vi "WPI_CANTalonSRX_Open.vi"(6 "Invert":bool, 8 "error in":errorcluster, 9 "Master Device Number":u8, 10 "Device Number":u8, 11 "Control Mode":T1) -> (0 "error out":errorcluster, 3 "CAN Talon SRX Ref":T2={"DeviceStatus"={"status"=FALSE, "code"=0, "source"=""}, "Type"=enum."PWM", "PWM"={"PWM Channel"=enum."PWM 1", "DeadBand"={"Name"="", "maxPositivePwm"=0, "minPositivePwm"=0, "centerPwm"=0, "maxNegativePwm"=0, "minNegativePwm"=0, "angularRange"=0}}, "CAN"={"Device Number"=0, "SetOutput VI Ref"=variant(enum8{"Percent VBus", "Current", "Speed", "Position", "Voltage"} enum."Percent VBus"), "GetOutput VI Ref"=variant(refnum<k1> refnum), "Enable VI Ref"=variant(dbl 12.0), "Disable VI Ref"=variant(enum8{"Percent VBus", "Speed", "Position", "Slave", "Unchanged / Invalid", "Voltage Compensation", "Current", "Motion Profile"} enum."Percent VBus"), "Data"=variant}, "Invert"=FALSE})   [LabVIEW 2016]
doc: "Read status information from a CAN Jaguar.\n\nThis VI allows you to specify which parts of the status you care about so that you do not waste CAN bus bandwidth. Use this VI to read status <B>On Demand</B> or status that is already received on a <B>Periodic Status Channel</B>.\n\nAll outputs are in engineering units (Volts, Amps, degrees Celsius, Rotations, and Rotations per Minute)\n\nSticky outputs are faults or limits that have occurred since the last time they were read, but may not be the current condition."
uses:
  <vilib>/Rock Robotics/WPI/MotorControl/WPI_MotorControlDeviceRef.ctl
  <vilib>/Rock Robotics/WPI/MotorControl/WPI_MotorControlType.ctl
  <vilib>/Rock Robotics/SystemInterfaces/DIO/FPGA_DIOPWMChannel.ctl
  <vilib>/Rock Robotics/WPI/PWM/WPI_PWMDeadband.ctl
  WPI_CANTalonSRX_APIControlMode.ctl
  WPI_CANTalonSRX_GlobalOps.ctl
  <vilib>/Rock Robotics/SystemInterfaces/NetworkCommunication/NetComm_UsageReport_ResourceType.ctl
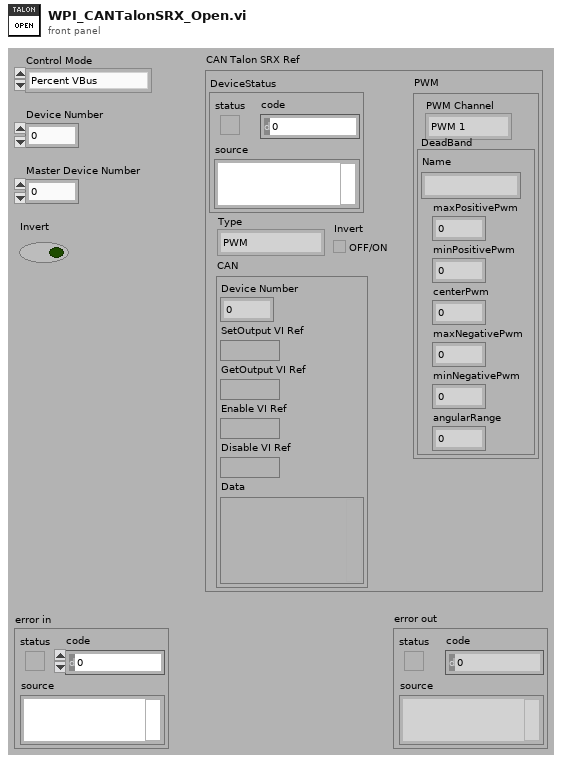
[diagram p1: front panel]
types:
  T1 = typedef "WPI_CANTalonSRX_APIControlMode.ctl" = enum8{"Percent VBus", "Speed", "Position", "Slave", "Unchanged / Invalid", "Voltage Compensation", "Current", "Motion Profile", "Motion Magic"}
  T2 = typedef "WPI_MotorControlDeviceRef.ctl" = cluster{"DeviceStatus":errorcluster, "Type":T3, "PWM":cluster{"PWM Channel":T4, "DeadBand":T5}, "CAN":cluster{"Device Number":u8, "SetOutput VI Ref":variant, "GetOutput VI Ref":variant, "Enable VI Ref":variant, "Disable VI Ref":variant, "Data":variant}, "Invert":bool}
  T3 = typedef "WPI_MotorControlType.ctl" = enum16{"PWM", "CAN"}
  T4 = typedef "FPGA_DIOPWMChannel.ctl" = enum8{"PWM 0", "PWM 1", "PWM 2", "PWM 3", "PWM 4", "PWM 5", "PWM 6", "PWM 7", "PWM 8", "PWM 9", "PWM MXP 0", "PWM MXP 1", "PWM MXP 2", "PWM MXP 3", "PWM MXP 4", "PWM MXP 5", "PWM MXP 6", "PWM MXP 7", "PWM MXP 8", "PWM MXP 9", "Invalid"}
  T5 = typedef "WPI_PWMDeadband.ctl" = cluster{"Name":string, "maxPositivePwm":i32, "minPositivePwm":i32, "centerPwm":i32, "maxNegativePwm":i32, "minNegativePwm":i32, "angularRange":u16}
  T6 = typedef "WPI_CANTalonSRX_GlobalOps.ctl" = enum16{"Read For Send", "Write After Receive General", "Write After Receive Feedback", "Write After Receive Encoder", "Write After Receive Ain", "Write Error", "Get All", "Set Output", "Set Mode", "Set Master ID", "Set Brake Mode", "Set Reverse Feedback Sensor", "Set Reverse Closed Loop Output", "Set Override Limits", "Set Forward Limit Enabled", "Set Reverse Limit Enabled", "Set Feedback Select", "Set Profile Select", "Set Throttle Ramp Rate", "Disable", "Set Enc Codes Per Rev", "Set Num Pot Turns", "Set Control Frame Rate", "Enable Legacy Control", "Write After Receive Pulse Width", "Set Enable Frame Rate", "Write After Receive Motion Profile", "Set Motion Profile Flow Control", "Set Motion Profile Control Frame Rate", "Set Current Limit Enable"}
  T7 = typedef "NetComm_UsageReport_ResourceType.ctl" = enum8{"Controller", "Module", "Language", "CANPlugin", "Accelerometer", "ADXL345", "AnalogChannel", "AnalogTrigger", "AnalogTriggerOutput", "CANJaguar", "Compressor", "Counter", "Dashboard", "DigitalInput", "DigitalOutput", "DriverStationCIO", "DriverStationEIO", "DriverStationLCD", "Encoder", "GearTooth", "Gyro", "I2C", "Framework", "Jaguar", "Joystick", "Kinect", "KinectStick", "PIDController", "Preferences", "PWM", "Relay", "RobotDrive", "SerialPort", "Servo", "Solenoid", "SPI", "Task", "Ultrasonic", "Victor", "Button", "Command", "AxisCamera", "PCVideoServer", "SmartDashboard", "Talon", "HiTechnicColorSensor", "HiTechnicAccel", "HiTechnicCompass", "SRF08", "AnalogOutput", "Victor SP", "Talon SRX", "CAN Talon SRX", "ADXL362 Accel", "ADXRS450 Gyro", "Rev SPARK", "Mindsensors SD540", "Digital Filter", "ADIS16448", "PDP", "PCM", "PigeonIMU"}
  T8 = cluster{"Control Mode":T1, "Encoder Initial Position":dbl, "MaxVout":dbl}
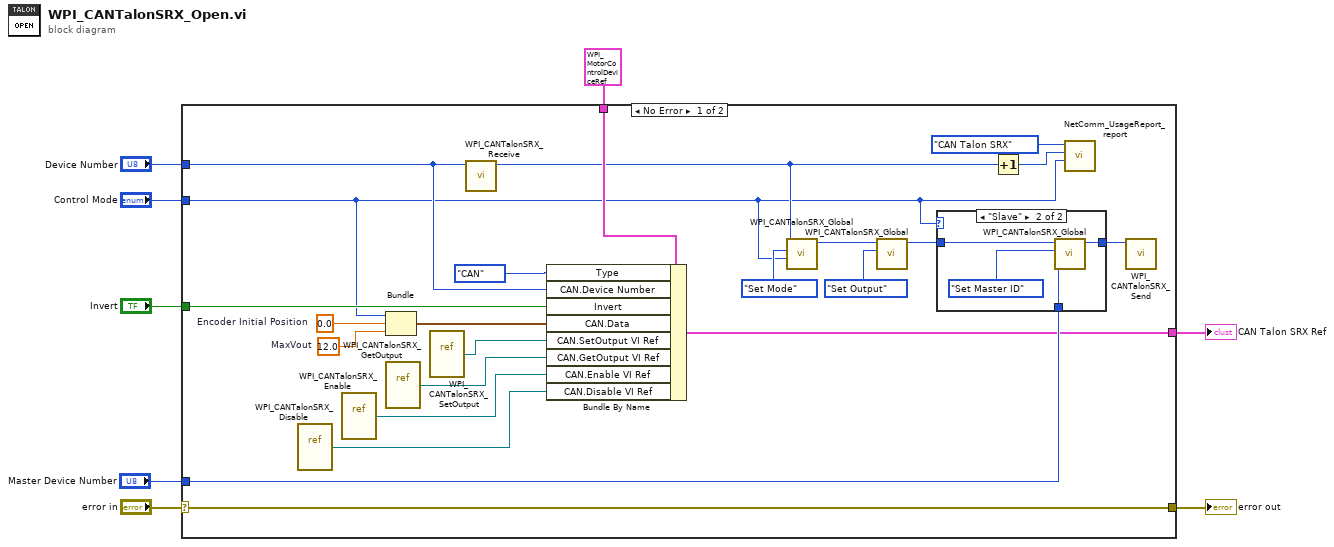
[diagram p0: block diagram]
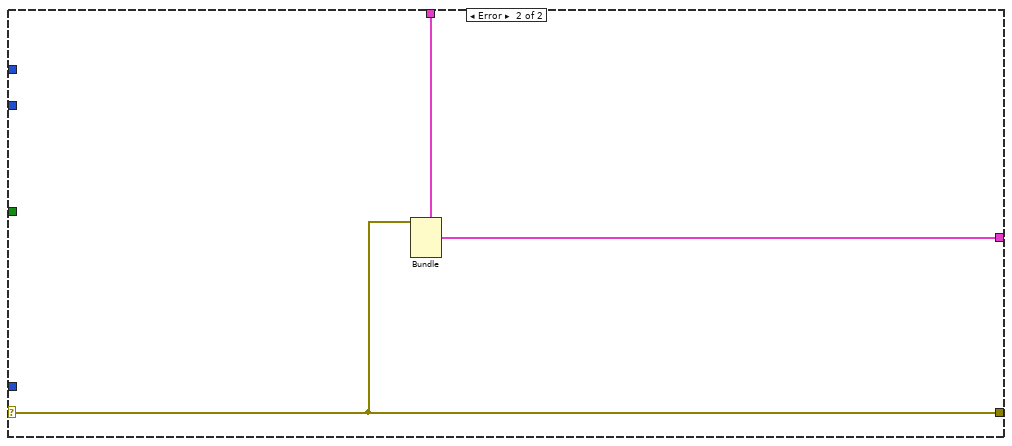
[diagram p3: hidden frame]
diagram:
  n1 = case shown="No Error" "error in" {
    selector: "error in" -> [w14 w37]
    tunnel: [w14 w37] -> w8
    tunnel: "Invert" -> [w22 _]
    tunnel: T2 {"DeviceStatus"={"status"=FALSE, "code"=0, "source"=""}, "Type"=enum."CAN", "PWM"={"PWM Channel"=enum."PWM 1", "DeadBand"={"Name"="", "maxPositivePwm"=0, "minPositivePwm"=0, "centerPwm"=0, "maxNegativePwm"=0, "minNegativePwm"=0, "angularRange"=0}}, "CAN"={"Device Number"=0, "SetOutput VI Ref"=variant(refnum<vi> refnum), "GetOutput VI Ref"=variant(refnum<vi> refnum), "Enable VI Ref"=variant(refnum<vi> refnum), "Disable VI Ref"=variant(refnum<vi> refnum), "Data"=variant(cluster{"Control Mode":enum8{"Percent VBus", "Speed", "Position", "Slave", "Unchanged / Invalid", "Voltage Compensation", "Current", "Motion Profile"}, "Encoder Initial Position":dbl, "MaxVout":dbl} {"Control Mode"=enum."Percent VBus", "Encoder Initial Position"=0.0, "MaxVout"=12.0})}, "Invert"=FALSE} ("CAN Talon SRX Ref") -> [w30 w39]
    tunnel: "Device Number" -> [w23 _]
    tunnel: "Control Mode" -> [w17 _]
    tunnel: "Master Device Number" -> [w13 _]
    tunnel: [w12 w38] -> w2
    frame No Error {
      w25 = 12.0  # MaxVout
      w24 = 0.0  # Encoder Initial Position
      n2 = vi-ref "WPI_CANTalonSRX_Disable.vi"() -> (w9:refnum<vi>)
      n3 = vi-ref "WPI_CANTalonSRX_Enable.vi"() -> (w10:refnum<vi>)
      n4 = Bundle("Control Mode"=w17, "Encoder Initial Position"=w24, "MaxVout"=w25) -> (w21:T8)  [unwired: 1 in]
      n5 = vi-ref "WPI_CANTalonSRX_GetOutput.vi"() -> (w11:refnum<vi>)
      n6 = vi-ref "WPI_CANTalonSRX_SetOutput.vi"() -> (w28:refnum<vi>)
      n7 = call "WPI_CANTalonSRX_Receive.vi"("Device ID (0)"=w23) -> ("Device ID"=w18:u8)  [unwired: 10 in]
      n8 = Bundle By Name(cluster=w30, "Type"=WPI_MotorControlType."CAN", "CAN.Device Number"=w23, "Invert"=w22, "CAN.Data"=w21, "CAN.SetOutput VI Ref"=w28, "CAN.GetOutput VI Ref"=w11, "CAN.Enable VI Ref"=w10, "CAN.Disable VI Ref"=w9) -> (w12:T2)
      n9 = call "WPI_CANTalonSRX_Global.vi"("Control Mode"=w17, "Operation"=WPI_CANTalonSRX_GlobalOps."Set Mode", "Device ID (0)"=w18) -> ("Device ID Out"=w19:u8)  [unwired: 6 in, 2 out]
      n10 = call "WPI_CANTalonSRX_Global.vi"("Operation"=WPI_CANTalonSRX_GlobalOps."Set Output", "Device ID (0)"=w19) -> ("Device ID Out"=w16:u8)  [unwired: 7 in, 2 out]
      n11 = case shown="\"Slave\"" w17 {
        tunnel: w16 -> [w32 w36]
        tunnel: [w32 w34] -> w15
        tunnel: w13 -> [_ w33]
        frame Default {
        }
        frame "Slave" {
          n12 = call "WPI_CANTalonSRX_Global.vi"("Set Number"=w33, "Operation"=WPI_CANTalonSRX_GlobalOps."Set Master ID", "Device ID (0)"=w36) -> ("Device ID Out"=w34:u8)  [unwired: 6 in, 2 out]
        }
      }
      n13 = Increment(x=w18) -> (x+1=w27:u8)
      n14 = call <vilib>:"NetComm_UsageReport_report.vi"("Context"=w17, "Instance Number"=w27, "Resource Type"=NetComm_UsageReport_ResourceType."CAN Talon SRX") -> ()  [unwired: 9 in]
      n15 = call "WPI_CANTalonSRX_Send.vi"("Device ID (0)"=w15) -> ()  [unwired: 10 in, 1 out]
    }
    frame Error {
      n16 = Bundle(cluster=w39, "DeviceStatus"=w37) -> (w38:T2)  [unwired: 4 in]
    }
  }
  "CAN Talon SRX Ref" <- w2
  "error out" <- w8
